vi "get stack parameters for qualification round.vi"(6 "cnt":i32, 7 "Type":enum16{"Z", "I", "O", "S", "L", "J", "T", "N"}(ring)) -> (0 "ang2":i8, 1 "ang1":i8, 2 "c2":i16, 3 "c1":i16, 4 "row":i8)   [LabVIEW 2018]
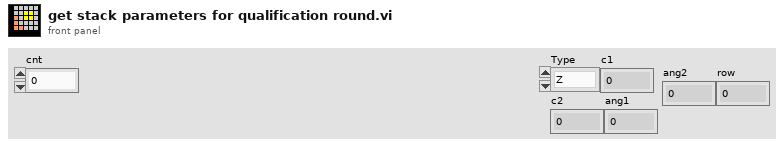
[diagram p1: front panel]
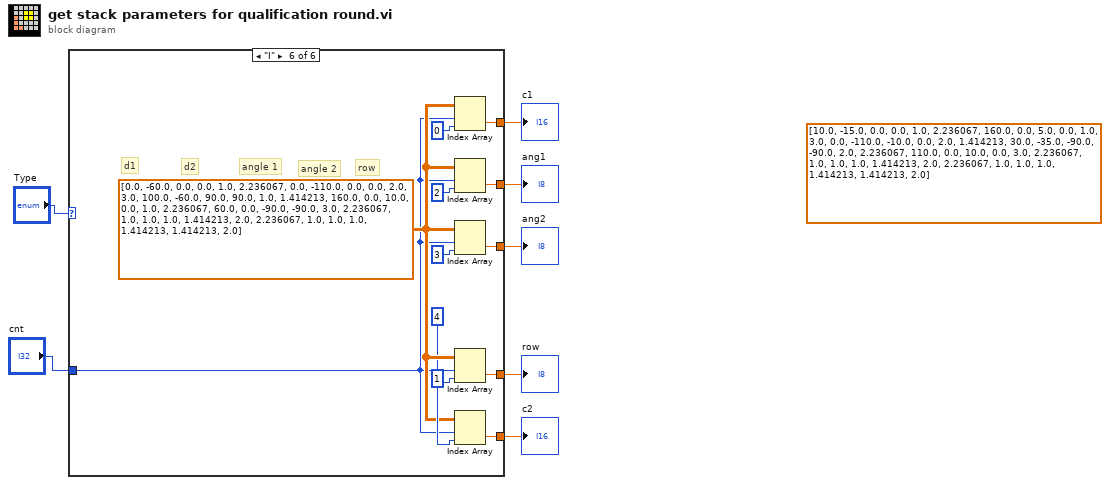
[diagram p0: block diagram]
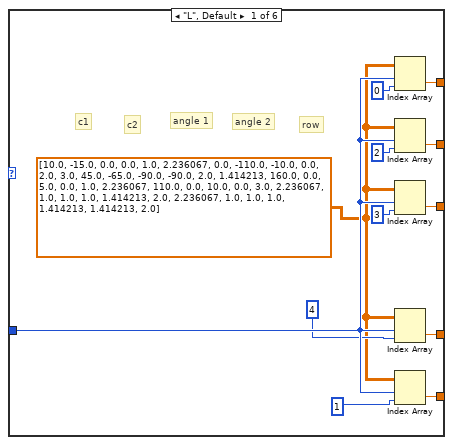
[diagram p2: hidden frame]
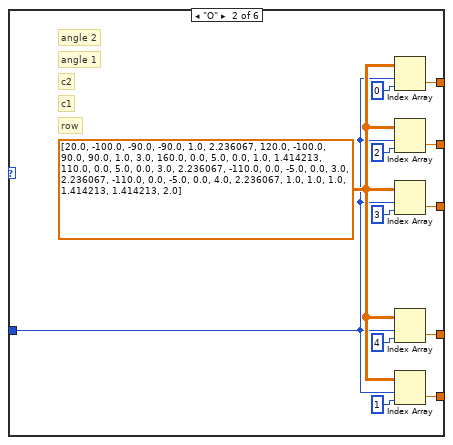
[diagram p3: hidden frame]
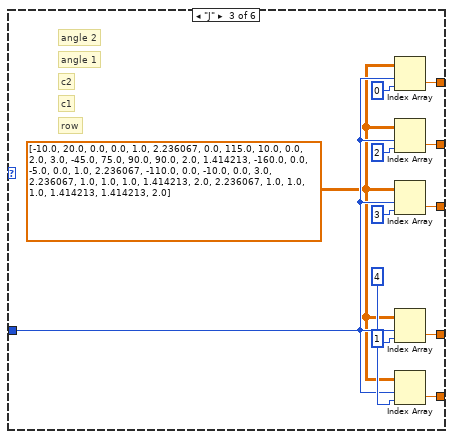
[diagram p4: hidden frame]
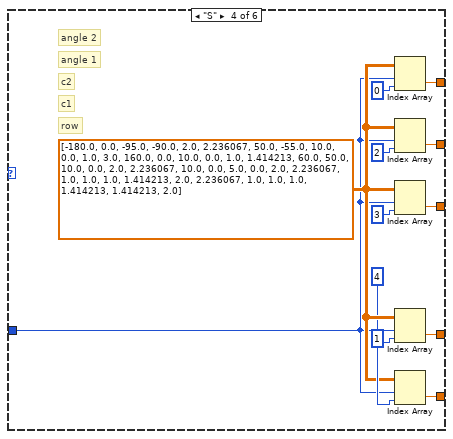
[diagram p5: hidden frame]
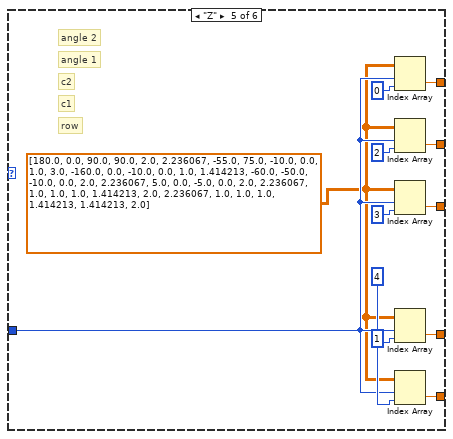
[diagram p6: hidden frame]
diagram:
  (unwired) dbl[][] [[10.0, -15.0, 0.0, 0.0, 1.0, 2.236067], [160.0, 0.0, 5.0, 0.0, 1.0, 3.0], [0.0, -110.0, -10.0, 0.0, 2.0, 1.414213], [30.0, -35.0, -90.0, -90.0, 2.0, 2.236067], [110.0, 0.0, 10.0, 0.0, 3.0, 2.236067], [1.0, 1.0, 1.0, 1.414213, 2.0, 2.236067], [1.0, 1.0, 1.0, 1.414213, 1.414213, 2.0]] ("Descriptors")
  n1 = case shown="\"I\"" "Type" {
    tunnel: "cnt" -> [w11 w22 w35 w46 w59 w70]
    tunnel: [w18 w30 w42 w54 w66 w78] -> w5
    tunnel: [w16 w28 w40 w52 w64 w76] -> w4
    tunnel: [w14 w26 w38 w50 w62 w74] -> w3
    tunnel: [w13 w25 w37 w49 w61 w73] -> w2
    tunnel: [w12 w23 w36 w47 w60 w71] -> w1
    frame "L", Default {
      w8 = dbl[][] [[10.0, -15.0, 0.0, 0.0, 1.0, 2.236067], [0.0, -110.0, -10.0, 0.0, 2.0, 3.0], [45.0, -65.0, -90.0, -90.0, 2.0, 1.414213], [160.0, 0.0, 5.0, 0.0, 1.0, 2.236067], [110.0, 0.0, 10.0, 0.0, 3.0, 2.236067], [1.0, 1.0, 1.0, 1.414213, 2.0, 2.236067], [1.0, 1.0, 1.0, 1.414213, 1.414213, 2.0]] ("Descriptors")
      # "row"
      # "angle 2"
      # "angle 1"
      # "c2"
      # "c1"
      n2 = Index Array(array=w8, index (row)=w11, index (col)=0 ("disabled index (col)")) -> (element=w18:dbl)
      n3 = Index Array(array=w8, index (row)=w11, index (col)=2 ("disabled index (col)")) -> (element=w14:dbl)
      n4 = Index Array(array=w8, index (row)=w11, index (col)=3 ("disabled index (col)")) -> (element=w13:dbl)
      n5 = Index Array(array=w8, index (row)=w11, index (col)=4 ("disabled index (col)")) -> (element=w12:dbl)
      n6 = Index Array(array=w8, index (row)=w11, index (col)=1 ("disabled index (col)")) -> (element=w16:dbl)
    }
    frame "O" {
      w24 = dbl[][] [[20.0, -100.0, -90.0, -90.0, 1.0, 2.236067], [120.0, -100.0, 90.0, 90.0, 1.0, 3.0], [160.0, 0.0, 5.0, 0.0, 1.0, 1.414213], [110.0, 0.0, 5.0, 0.0, 3.0, 2.236067], [-110.0, 0.0, -5.0, 0.0, 3.0, 2.236067], [-110.0, 0.0, -5.0, 0.0, 4.0, 2.236067], [1.0, 1.0, 1.0, 1.414213, 1.414213, 2.0]] ("Descriptors")
      # "row"
      # "angle 2"
      # "angle 1"
      # "c2"
      # "c1"
      n7 = Index Array(array=w24, index (row)=w22, index (col)=0 ("disabled index (col)")) -> (element=w30:dbl)
      n8 = Index Array(array=w24, index (row)=w22, index (col)=2 ("disabled index (col)")) -> (element=w26:dbl)
      n9 = Index Array(array=w24, index (row)=w22, index (col)=3 ("disabled index (col)")) -> (element=w25:dbl)
      n10 = Index Array(array=w24, index (row)=w22, index (col)=4 ("disabled index (col)")) -> (element=w23:dbl)
      n11 = Index Array(array=w24, index (row)=w22, index (col)=1 ("disabled index (col)")) -> (element=w28:dbl)
    }
    frame "J" {
      w32 = dbl[][] [[-10.0, 20.0, 0.0, 0.0, 1.0, 2.236067], [0.0, 115.0, 10.0, 0.0, 2.0, 3.0], [-45.0, 75.0, 90.0, 90.0, 2.0, 1.414213], [-160.0, 0.0, -5.0, 0.0, 1.0, 2.236067], [-110.0, 0.0, -10.0, 0.0, 3.0, 2.236067], [1.0, 1.0, 1.0, 1.414213, 2.0, 2.236067], [1.0, 1.0, 1.0, 1.414213, 1.414213, 2.0]] ("Descriptors")
      # "row"
      # "angle 2"
      # "angle 1"
      # "c2"
      # "c1"
      n12 = Index Array(array=w32, index (row)=w35, index (col)=0 ("disabled index (col)")) -> (element=w42:dbl)
      n13 = Index Array(array=w32, index (row)=w35, index (col)=2 ("disabled index (col)")) -> (element=w38:dbl)
      n14 = Index Array(array=w32, index (row)=w35, index (col)=3 ("disabled index (col)")) -> (element=w37:dbl)
      n15 = Index Array(array=w32, index (row)=w35, index (col)=4 ("disabled index (col)")) -> (element=w36:dbl)
      n16 = Index Array(array=w32, index (row)=w35, index (col)=1 ("disabled index (col)")) -> (element=w40:dbl)
    }
    frame "S" {
      w48 = dbl[][] [[-180.0, 0.0, -95.0, -90.0, 2.0, 2.236067], [50.0, -55.0, 10.0, 0.0, 1.0, 3.0], [160.0, 0.0, 10.0, 0.0, 1.0, 1.414213], [60.0, 50.0, 10.0, 0.0, 2.0, 2.236067], [10.0, 0.0, 5.0, 0.0, 2.0, 2.236067], [1.0, 1.0, 1.0, 1.414213, 2.0, 2.236067], [1.0, 1.0, 1.0, 1.414213, 1.414213, 2.0]] ("Descriptors")
      # "row"
      # "angle 2"
      # "angle 1"
      # "c2"
      # "c1"
      n17 = Index Array(array=w48, index (row)=w46, index (col)=0 ("disabled index (col)")) -> (element=w54:dbl)
      n18 = Index Array(array=w48, index (row)=w46, index (col)=2 ("disabled index (col)")) -> (element=w50:dbl)
      n19 = Index Array(array=w48, index (row)=w46, index (col)=3 ("disabled index (col)")) -> (element=w49:dbl)
      n20 = Index Array(array=w48, index (row)=w46, index (col)=4 ("disabled index (col)")) -> (element=w47:dbl)
      n21 = Index Array(array=w48, index (row)=w46, index (col)=1 ("disabled index (col)")) -> (element=w52:dbl)
    }
    frame "Z" {
      w56 = dbl[][] [[180.0, 0.0, 90.0, 90.0, 2.0, 2.236067], [-55.0, 75.0, -10.0, 0.0, 1.0, 3.0], [-160.0, 0.0, -10.0, 0.0, 1.0, 1.414213], [-60.0, -50.0, -10.0, 0.0, 2.0, 2.236067], [5.0, 0.0, -5.0, 0.0, 2.0, 2.236067], [1.0, 1.0, 1.0, 1.414213, 2.0, 2.236067], [1.0, 1.0, 1.0, 1.414213, 1.414213, 2.0]] ("Descriptors")
      # "row"
      # "angle 2"
      # "angle 1"
      # "c2"
      # "c1"
      n22 = Index Array(array=w56, index (row)=w59, index (col)=0 ("disabled index (col)")) -> (element=w66:dbl)
      n23 = Index Array(array=w56, index (row)=w59, index (col)=2 ("disabled index (col)")) -> (element=w62:dbl)
      n24 = Index Array(array=w56, index (row)=w59, index (col)=3 ("disabled index (col)")) -> (element=w61:dbl)
      n25 = Index Array(array=w56, index (row)=w59, index (col)=4 ("disabled index (col)")) -> (element=w60:dbl)
      n26 = Index Array(array=w56, index (row)=w59, index (col)=1 ("disabled index (col)")) -> (element=w64:dbl)
    }
    frame "I" {
      w72 = dbl[][] [[0.0, -60.0, 0.0, 0.0, 1.0, 2.236067], [0.0, -110.0, 0.0, 0.0, 2.0, 3.0], [100.0, -60.0, 90.0, 90.0, 1.0, 1.414213], [160.0, 0.0, 10.0, 0.0, 1.0, 2.236067], [60.0, 0.0, -90.0, -90.0, 3.0, 2.236067], [1.0, 1.0, 1.0, 1.414213, 2.0, 2.236067], [1.0, 1.0, 1.0, 1.414213, 1.414213, 2.0]] ("Descriptors")
      # "row"
      # "angle 2"
      # "angle 1"
      # "d2"
      # "d1"
      n27 = Index Array(array=w72, index (row)=w70, index (col)=0 ("disabled index (col)")) -> (element=w78:dbl)
      n28 = Index Array(array=w72, index (row)=w70, index (col)=2 ("disabled index (col)")) -> (element=w74:dbl)
      n29 = Index Array(array=w72, index (row)=w70, index (col)=3 ("disabled index (col)")) -> (element=w73:dbl)
      n30 = Index Array(array=w72, index (row)=w70, index (col)=4 ("disabled index (col)")) -> (element=w71:dbl)
      n31 = Index Array(array=w72, index (row)=w70, index (col)=1 ("disabled index (col)")) -> (element=w76:dbl)
    }
  }
  "c1" <- w5
  "c2" <- w4
  "ang1" <- w3
  "ang2" <- w2
  "row" <- w1
